vi "Macro_Text Array to Instruction and Argument array.vi"(8 "Error In":errorcluster, 11 "Macro Array IN":string[](array[string])) -> (0 "Error Out":errorcluster, 2 "Argument List (Txt)":string[](array[string]), 3 "Action List (Txt)":string[](array[string]))   [LabVIEW 2012]
doc: "SciScan 1.2 160622"
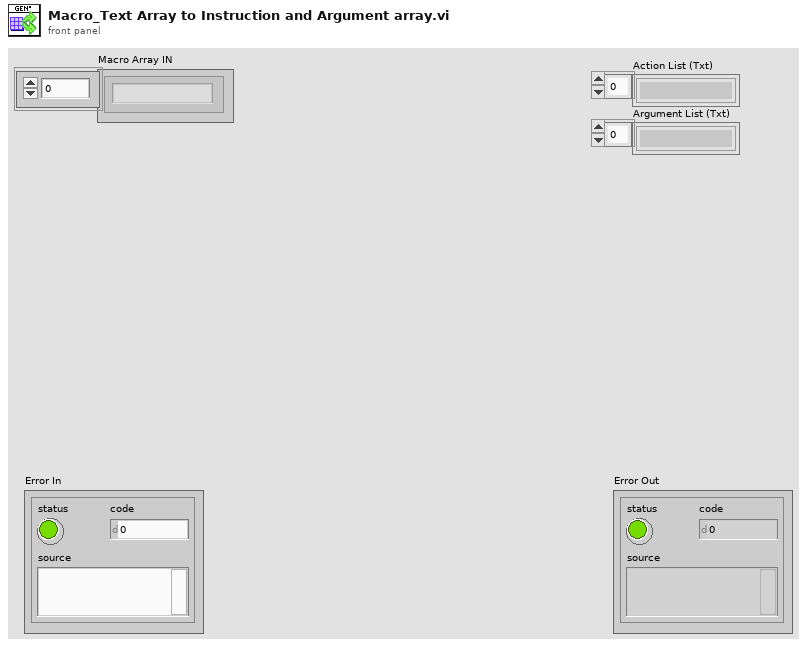
[diagram p1: front panel]
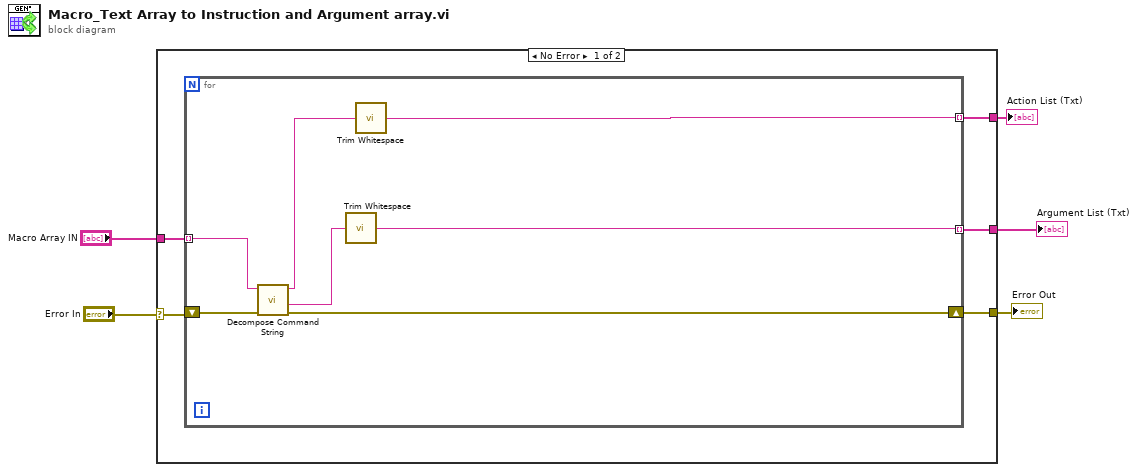
[diagram p0: block diagram]
diagram:
  n1 = case shown="No Error" "Error In" {
    selector: "Error In" -> [w9 w18]
    tunnel: "Macro Array IN" -> [w10 _]
    tunnel: [w8 _] -> w3
    tunnel: [w7 _] -> w2
    tunnel: [w6 w18] -> w1
    frame No Error {
      n2 = for {
        tunnel: w10 -> [w17] mode=indexing
        tunnel: [w11] -> w8 mode=indexing
        tunnel: [w12] -> w7 mode=indexing
        shift-right: [w15] -> w6
        shift-left: w9 -> [w16]
        n3 = call "Decompose Command String.vi"("Error In"=w16, "Command IN"=w17) -> ("Error Out"=w15:errorcluster, "Parameter Text"=w13:string, "Action"=w14:string)  [unwired: 6 in, 1 out]
        n4 = call <vilib>:"Trim Whitespace.vi"("string"=w13) -> ("trimmed string"=w12:string)  [unwired: 1 in]
        n5 = call <vilib>:"Trim Whitespace.vi"("string"=w14) -> ("trimmed string"=w11:string)  [unwired: 1 in]
      }
    }
    frame Error {
    }
  }
  "Error Out" <- w1
  "Action List (Txt)" <- w3
  "Argument List (Txt)" <- w2
